vi "Tester.vi"() -> ()   [LabVIEW 2023, in "Error Manager.lvlib" / "New Error Dialogue GUI.lvlib" / "MHL Queue.lvlib"]
doc: "Tester"
uses:
  MHL Queue.lvlib
  Command (enum).ctl
panel:
  out "EHL iteration":i32
  out "MHL iteration":i32
  in  "Exit Tester":bool
  in  "Command Data":string="This is an example of command data. The command data is a variant, so it can carry any data type."
  in  "Command to send":T1
  in  "Send Command":bool
  out "Queue Name":string
  out "No. Of Elements in Queue":i32
  out "Data Received":variant
  out "Command Received":T1
  out "Error Out":errorcluster
  # "Tester"
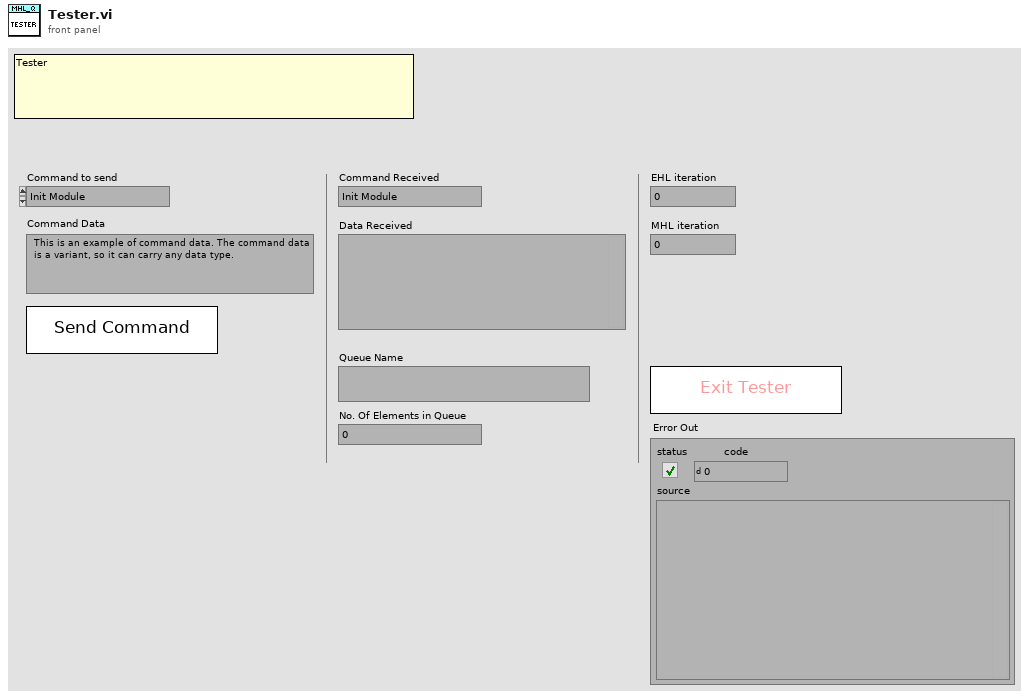
[diagram p1: front panel]
types:
  T1 = typedef "Error Manager.lvlib/New Error Dialogue GUI.lvlib/MHL Queue.lvlib/Command (enum).ctl" = enum16{"Init Module", "Close Module", "Handle Local Error", "OK Button Pressed"}
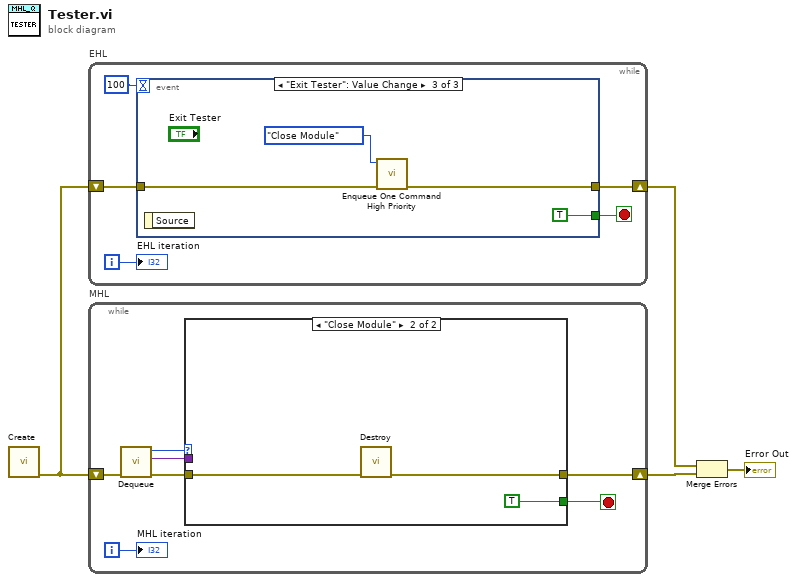
[diagram p0: block diagram]
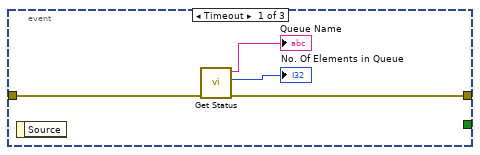
[diagram p2: hidden frame]
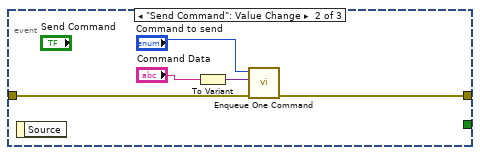
[diagram p3: hidden frame]
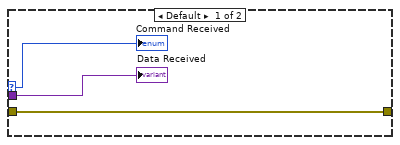
[diagram p4: hidden frame]
diagram:
  n1 = call "Create.vi"() -> ("error out"=w4:errorcluster)  [unwired: 11 in]
  n2 = while "EHL" {
    shift-right: [w7] -> w3
    shift-left: w4 -> [w8]
    i -> [w5]
    stop <- w6 stop-if-true
    n3 = event shown="[2] \"Exit Tester\": Value Change" {
      selector: _ -> [_ _ _]
      dyn-events: _ -> [_ _ _]
      timeout: 100 -> [_ _ _]
      tunnel: w8 -> [w13 w18 w22]
      tunnel: [w12 w17 w21] -> w7
      tunnel: [_ _ TRUE] -> w6
      event Timeout {
        n4 = event-data() -> ()  [unwired: 1 in, 1 out]
        n5 = call "Get Status.vi"("error in (no error)"=w13) -> ("error out"=w12:errorcluster, "No. Of Elements in Queue"=→"No. Of Elements in Queue":i32, "Queue Name"=→"Queue Name":string)  [unwired: 8 in]
      }
      event "Send Command": Value Change {
        n6 = event-data() -> ()  [unwired: 1 in, 1 out]
        n7 = To Variant(anything="Command Data") -> (Variant=w14:variant)
        n8 = call "Enqueue One Command.vi"("error in (no error)"=w18, "Data"=w14, "Command"="Command to send") -> ("error out"=w17:errorcluster)  [unwired: 8 in]
      }
      event "Exit Tester": Value Change {
        n9 = event-data() -> ()  [unwired: 1 in, 1 out]
        n10 = call "Enqueue One Command High Priority.vi"("error in (no error)"=w22, "Command"=Command_(enum)."Close Module") -> ("error out"=w21:errorcluster)  [unwired: 9 in]
      }
    }
    "EHL iteration" <- w5
  }
  n11 = while "MHL" {
    shift-right: [w27] -> w2
    shift-left: w4 -> [w29]
    i -> [w23]
    stop <- w24 stop-if-true
    n12 = call "Dequeue.vi"("error in (no error)"=w29) -> ("error out"=w28:errorcluster, "Data"=w25:variant, "Command"=w26:T1)  [unwired: 8 in]
    n13 = case shown="\"Close Module\"" w26 {
      selector: w26 -> [w31 _]
      tunnel: w28 -> [w32 w34]
      tunnel: [w32 w33] -> w27
      tunnel: w25 -> [w30 _]
      tunnel: [_ TRUE] -> w24
      frame Default {
        "Command Received" <- w31
        "Data Received" <- w30
      }
      frame "Close Module" {
        n14 = call "Destroy.vi"("error in (no error)"=w34) -> ("error out"=w33:errorcluster)  [unwired: 8 in, 2 out]
      }
    }
    "MHL iteration" <- w23
  }
  n15 = Merge Errors(w3, w2) -> (→"Error Out":errorcluster)
